vi "OC_SC_Detection.vi"() -> (2 "Open Loop Channels Array":bool[](array[boolean]), 3 "Short Circuit Channels Array":bool[](array[boolean]))   [LabVIEW 2017, in "BOP_VibAPI_2.lvlib"]
uses:
  <vilib>/addons/InsightCM/Devices/Shared/Cms/Fpga/Acquisition/source/subVIs/VibAPI_2/BOP_VibAPI_2.lvlib
  <vilib>/rvi/eio/common/nirviEmuTemplateMethod_errors.vi
  <vilib>/eio/EIOMethodNode/EIOMethodNode.xnode
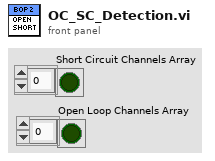
[diagram p1: front panel]
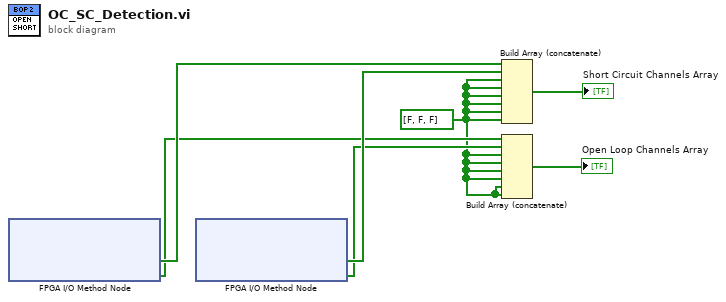
[diagram p0: block diagram]
diagram:
  w1 = bool[] [FALSE, FALSE, FALSE] ("array")
  n1 = xnode "FPGA I/O Method Node"() -> ("Short Circuit"=w7:bool[], "Open Loop"=w5:bool[])  [unwired: 1 in, 1 out]
  n2 = xnode "FPGA I/O Method Node"() -> ("Short Circuit"=w6:bool[], "Open Loop"=w4:bool[])  [unwired: 1 in, 1 out]
  n3 = Build Array (concatenate)(w7, w6, w1, w1, w1, w1, w1, w1) -> (→"Short Circuit Channels Array":bool[])
  n4 = Build Array (concatenate)(w5, w4, w1, w1, w1, w1, w1, w1) -> (→"Open Loop Channels Array":bool[])
